vi "4.5.vi"() -> ()   [LabVIEW 2017]
panel:
  in  "指定值":dbl
  out "执行次数":dbl
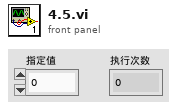
[diagram p1: front panel]
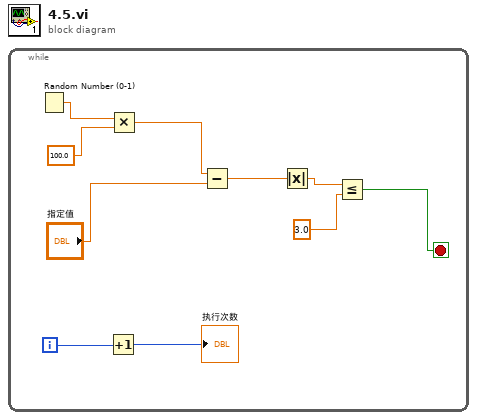
[diagram p0: block diagram]
diagram:
  n1 = while {
    i -> [w9]
    stop <- w1 stop-if-true
    n2 = Random Number (0-1)() -> (number: 0 to 1=w8:dbl)
    n3 = Increment(x=w9) -> (x+1=→"执行次数":i32)
    n4 = Multiply(x=w8, y=100.0) -> (x*y=w6:dbl)
    n5 = Subtract(x=w6, y="指定值") -> (x-y=w4:dbl)
    n6 = Absolute Value(x=w4) -> (abs(x)=w3:dbl)
    n7 = Less Or Equal?(x=w3, y=3.0) -> (x <= y?=w1:bool)
  }
